vi "Clock Divide by 2 with Data Valid.vi"(8 "Data Valid":bool, 11 "Reset?":bool) -> (3 "CLK/2":bool)   [LabVIEW 2012]
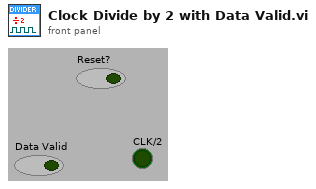
[diagram p1: front panel]
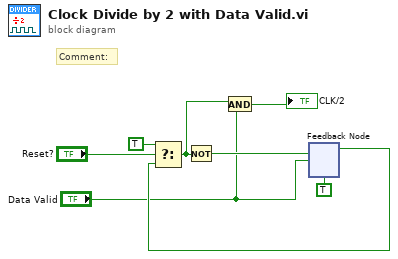
[diagram p0: block diagram]
diagram:
  # "Comment:"
  n1 = feedback #1(TRUE) -> (w4:bool)
  n2 = Select(t=TRUE, s="Reset?", f=w4) -> (s? t:f=w3:bool)
  n3 = Not(x=w3) -> (.not. x?=w5:bool)
  n4 = And(x=w3, y="Data Valid") -> (x .and. y?=→"CLK/2":bool)
  n5 = feedback-in #1(w5, "Data Valid") -> ()
